vi "IO_Waveforms_To_Spreadsheet(1D).vi"(4 "header? (write header:T)":bool=TRUE, 5 "delimiter (Tab)":string="\t", 6 "operation (0:open)":T1(ring), 7 "prompt":string="Choose file to write.", 8 "error in (no error)":errorcluster, 9 "multiple time columns? (single:F)":bool, 10 "waveforms":waveform(dbl)[](array[waveform]), 11 "file path (dialog if empty)":path) -> (0 "error out":errorcluster)   [LabVIEW 2012]
doc: "Converts a waveform to a text string and writes the string to a new byte stream file or appends the string to an existing file. Wire data to the <B>Waveform</B> input to determine the polymorphic instance to use or manually select the instance."
uses:
  <vilib>/Waveform/WDTOps.llb/WDT Get Waveform Time Array DBL.vi
panel:
  out "Array":string[](array[string])
  out "spreadsheet string":string
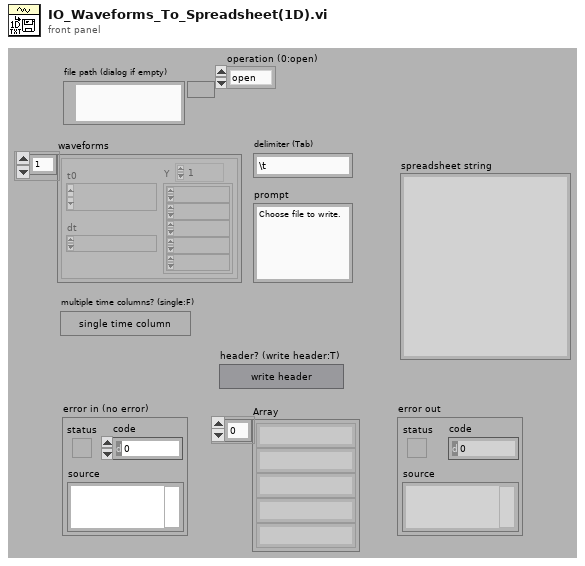
[diagram p1: front panel]
types:
  T1 = enum16{"open", "replace", "create", "open or create", "replace or create", "replace or create with confirmation"}
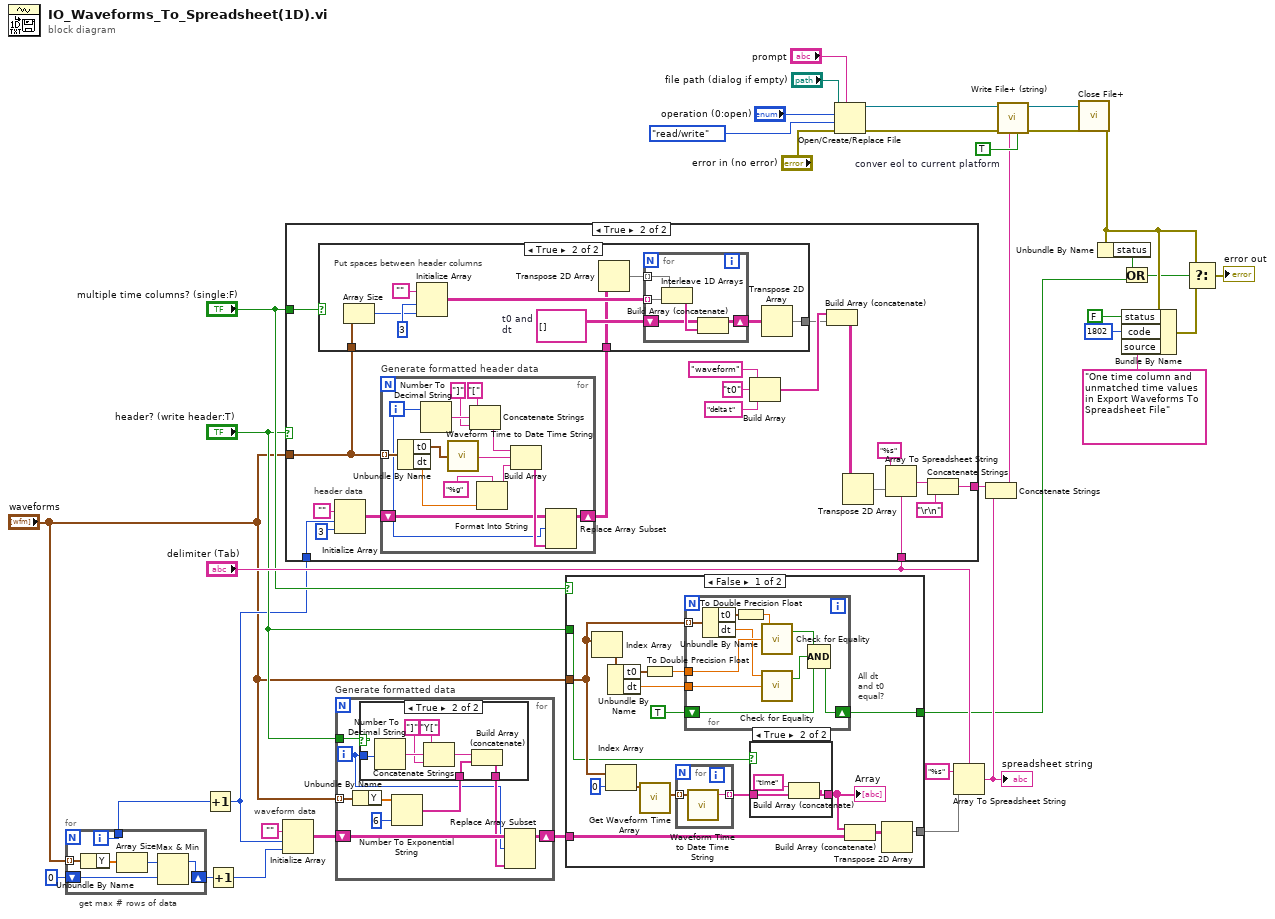
[diagram p0: block diagram]
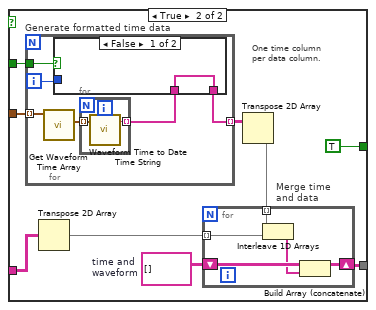
[diagram p3: hidden frame]
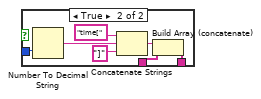
[diagram p4: hidden frame]
diagram:
  w33 = TRUE  # conver eol to current platform
  # "waveform data"
  # "get max # rows of data"
  n1 = for {
    tunnel: "waveforms" -> [w42] mode=indexing
    shift-right: [w38] -> w8
    shift-left: 0 -> [w39]
    tunnel: [w37] -> w6
    i -> [w37]
    n2 = Unbundle By Name(w42) -> ("Y"=w41:dbl[])
    n3 = Array Size(array=w41) -> (size(s)=w40:i32)
    n4 = Max & Min(x=w40, y=w39) -> (max(x,y)=w38:i32)  [unwired: 1 out]
  }
  n5 = Increment(x=w6) -> (x+1=w5:i32)
  n6 = Increment(x=w8) -> (x+1=w4:i32)
  n7 = Initialize Array("", w5, w4) -> (w7:string[][])
  n8 = case shown="True" "header? (write header:T)" {
    tunnel: "delimiter (Tab)" -> [_ w59]
    tunnel: "waveforms" -> [_ w53]
    tunnel: [_ w54] -> w24
    tunnel: "multiple time columns? (single:F)" -> [_ w51]
    tunnel: w5 -> [_ w44]
    frame False {
    }
    frame True {
      # "header data"
      n9 = Initialize Array("", w44, 3 ("dimension size")) -> (w43:string[][])
      n10 = for "Generate formatted header data" {
        tunnel: w53 -> [w84] mode=indexing
        shift-right: [w79] -> w49
        shift-left: w43 -> [w80]
        i -> [w78]
        n11 = Unbundle By Name(w84) -> ("t0"=w82:timestamp, "dt"=w89:dbl)
        n12 = Number To Decimal String(number=w78) -> (decimal integer string=w87:string)  [unwired: 1 in]
        n13 = call <vilib>:"Waveform Time to Date Time String.vi"("t0"=w82) -> ("String"=w90:string)
        n14 = Concatenate Strings("[", w87, "]") -> (w88:string)
        n15 = Format Into String(format string="%g" ("Format String"), w89) -> (resulting string=w91:string)  [unwired: 2 in, 1 out]
        n16 = Build Array(w88, w90, w91) -> (w81:string[])
        n17 = Replace Array Subset(array=w80, new element=w81, index (row)=w78) -> (w79:string[][])  [unwired: 1 in]
      }
      n18 = case shown="True" w51 {
        tunnel: w53 -> [_ w72]
        tunnel: [w62 w67] -> w50
        tunnel: w49 -> [w62 w66]
        frame False {
          # "Leave the header data alone"
        }
        frame True {
          w70 = string[][] []  # t0 and dt
          # "Put spaces between header columns"
          n19 = Array Size(array=w72) -> (size(s)=w63:i32)
          n20 = Initialize Array("", 3 ("Dimension Size"), w63) -> (w69:string[][])
          n21 = Transpose 2D Array(2D array=w66) -> (transposed array=w65:string[][])
          n22 = for {
            shift-right: [w74] -> w68
            shift-left: w70 -> [w75]
            tunnel: w69 -> [w77] mode=indexing
            tunnel: w65 -> [w73] mode=indexing
            n23 = Interleave 1D Arrays(w73, w77) -> (w76:string[])
            n24 = Build Array (concatenate)(w75, w76) -> (w74:string[][])
          }
          n25 = Transpose 2D Array(2D array=w68) -> (transposed array=w67:string[][])
        }
      }
      n26 = Build Array("waveform", "t0", "delta t") -> (w52:string[])
      n27 = Build Array (concatenate)(w52, w50) -> (w47:string[][])
      n28 = Transpose 2D Array(2D array=w47) -> (transposed array=w48:string[][])
      n29 = Array To Spreadsheet String(delimiter (Tab)=w59, array=w48, 3:"%s" ("format string")) -> (spreadsheet string=w56:string)
      n30 = Concatenate Strings(w56, "\r\n") -> (w54:string)
    }
  }
  n31 = for "Generate formatted data" {
    tunnel: "waveforms" -> [w98] mode=indexing
    tunnel: "header? (write header:T)" -> [w95]
    shift-right: [w96] -> w23
    shift-left: w7 -> [w97]
    i -> [w92]
    n32 = Unbundle By Name(w98) -> ("Y"=w100:dbl[])
    n33 = Number To Exponential String(number=w100, precision (6)=i16 6) -> (E-format string=w94:string[])  [unwired: 2 in]
    n34 = case shown="True" w95 {
      tunnel: w92 -> [_ w105]
      tunnel: w94 -> [w101 w103]
      tunnel: [w101 w102] -> w93
      frame False {
      }
      frame True {
        n35 = Number To Decimal String(number=w105) -> (decimal integer string=w108:string)  [unwired: 1 in]
        n36 = Concatenate Strings("Y[", w108, "]") -> (w104:string)
        n37 = Build Array (concatenate)(w104, w103) -> (w102:string[])
      }
    }
    n38 = Replace Array Subset(array=w97, new element=w93, index (row)=w92) -> (w96:string[][])  [unwired: 1 in]
  }
  n39 = case shown="False" "multiple time columns? (single:F)" {
    tunnel: "waveforms" -> [w113 w149]
    tunnel: w23 -> [w120 w147]
    tunnel: [w118 w143] -> w22
    tunnel: [w112 TRUE] -> w12
    tunnel: "header? (write header:T)" -> [w109 w141]
    frame False {
      # "One time column - check for equal dt and t0"
      # "All dt\nand t0\nequal?"
      n40 = Index Array(array=w113) -> (element=w117:waveform(dbl))  [unwired: 1 in]
      n41 = Index Array(array=w113, index=0 ("Index")) -> (element=w122:waveform(dbl))
      n42 = Unbundle By Name(w117) -> ("t0"=w111:timestamp, "dt"=w114:dbl)
      n43 = call-poly <vilib>:"Get Waveform Time Array.vi"("waveform in"=w122) -> ("X array"=w124:timestamp[])  [unwired: 9 in, 1 out]
      n44 = To Double Precision Float(number=w111) -> (double precision float=w115:dbl)
      n45 = for {
        tunnel: w124 -> [w139] mode=indexing
        tunnel: [w140] -> w121 mode=indexing
        n46 = call <vilib>:"Waveform Time to Date Time String.vi"("t0"=w139) -> ("String"=w140:string)
      }
      n47 = for {
        tunnel: w113 -> [w138] mode=indexing
        shift-right: [w133] -> w112
        shift-left: TRUE -> [w132]
        tunnel: w115 -> [w136]
        tunnel: w114 -> [w134]
        n48 = Unbundle By Name(w138) -> ("t0"=w129:timestamp, "dt"=w135:dbl)
        n49 = To Double Precision Float(number=w129) -> (double precision float=w137:dbl)
        n50 = call <vilib>:"Check for Equality.vi"("n2"=w136, "n1"=w137) -> ("equal?"=w130:bool)  [unwired: 1 in, 1 out]
        n51 = call <vilib>:"Check for Equality.vi"("n2"=w134, "n1"=w135) -> ("equal?"=w131:bool)  [unwired: 1 in, 1 out]
        n52 = Compound Arithmetic op=AND(w130, w131, w132) -> (w133:bool)
      }
      n53 = case shown="True" w109 {
        tunnel: w121 -> [w125 w128]
        tunnel: [w125 w127] -> w110
        frame False {
        }
        frame True {
          n54 = Build Array (concatenate)("time", w128) -> (w127:string[])
        }
      }
      "Array" <- w110
      n55 = Build Array (concatenate)(w110, w120) -> (w119:string[][])
      n56 = Transpose 2D Array(2D array=w119) -> (transposed array=w118:string[][])
    }
    frame True {
      w144 = string[][] []  # time and waveform
      # "One time column\nper data column."
      n57 = for "Generate formatted time data" {
        tunnel: [w155] -> w148 mode=indexing
        tunnel: w149 -> [w159] mode=indexing
        tunnel: w141 -> [w157]
        i -> [w158]
        n58 = call-poly <vilib>:"Get Waveform Time Array.vi"("waveform in"=w159) -> ("X array"=w160:timestamp[])  [unwired: 9 in, 1 out]
        n59 = for {
          tunnel: w160 -> [w169] mode=indexing
          tunnel: [w170] -> w156 mode=indexing
          n60 = call <vilib>:"Waveform Time to Date Time String.vi"("t0"=w169) -> ("String"=w170:string)
        }
        n61 = case shown="False" w157 {
          tunnel: w158 -> [_ w165]
          tunnel: w156 -> [w161 w163]
          tunnel: [w161 w162] -> w155
          frame False {
          }
          frame True {
            n62 = Number To Decimal String(number=w165) -> (decimal integer string=w168:string)  [unwired: 1 in]
            n63 = Concatenate Strings("time[", w168, "]") -> (w164:string)
            n64 = Build Array (concatenate)(w164, w163) -> (w162:string[])
          }
        }
      }
      n65 = Transpose 2D Array(2D array=w147) -> (transposed array=w146:string[][])
      n66 = Transpose 2D Array(2D array=w148) -> (transposed array=w145:string[][])
      n67 = for "Merge time\nand data" {
        tunnel: w146 -> [w153] mode=indexing
        tunnel: w145 -> [w152] mode=indexing
        shift-right: [w151] -> w143
        shift-left: w144 -> [w154]
        n68 = Interleave 1D Arrays(w152, w153) -> (w150:string[])
        n69 = Build Array (concatenate)(w154, w150) -> (w151:string[][])
      }
    }
  }
  n70 = Open/Create/Replace File(file path (use dialog)="file path (dialog if empty)", error in="error in (no error)", prompt="prompt", operation (0:open)="operation (0:open)", access (0:read/write)=enum16{"read/write", "read-only", "write-only"}."read/write") -> (refnum out=w27:refnum<file>, error out=w28:errorcluster)  [unwired: 1 in, 1 out]
  n71 = Array To Spreadsheet String(delimiter (Tab)="delimiter (Tab)", array=w22, 3:"%s" ("format (%.3f)")) -> (spreadsheet string=w26:string)
  "spreadsheet string" <- w26
  n72 = Concatenate Strings(w24, w26) -> (w25:string)
  n73 = call <vilib>:"Write File+ (string).vi"("convert eol? (no:F)"=w33, "string"=w25, "error in (no error)"=w28, "refnum"=w27) -> ("error out"=w36:errorcluster, "dup refnum"=w34:refnum<file>)  [unwired: 3 in, 1 out]
  n74 = call <vilib>:"Close File+.vi"("error in (no error)"=w36, "refnum"=w34) -> ("error out"=w19:errorcluster)  [unwired: 3 in, 2 out]
  n75 = Unbundle By Name(w19) -> ("status"=w18:bool)
  n76 = Or(x=w18, y=w12) -> (x .or. y?=w17:bool)
  n77 = Bundle By Name(cluster=w19, "status"=FALSE, "code"=1802, "source"="One time column and unmatched time values in Export Waveforms To Spreadsheet File") -> (w20:errorcluster)
  n78 = Select(t=w19, s=w17, f=w20) -> (s? t:f=→"error out":errorcluster)
